vi "AE Events.vi"(8 "error in (no error)":errorcluster, 10 "Event In":dbl, 11 "Action":enum16{"Init", "Get Event", "Set Event"}(ring)) -> (0 "error out":errorcluster, 2 "Event Out":dbl)   [LabVIEW 2013, in "main.lvlib"]
uses:
  main.lvlib
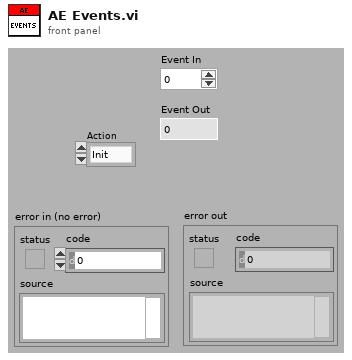
[diagram p1: front panel]
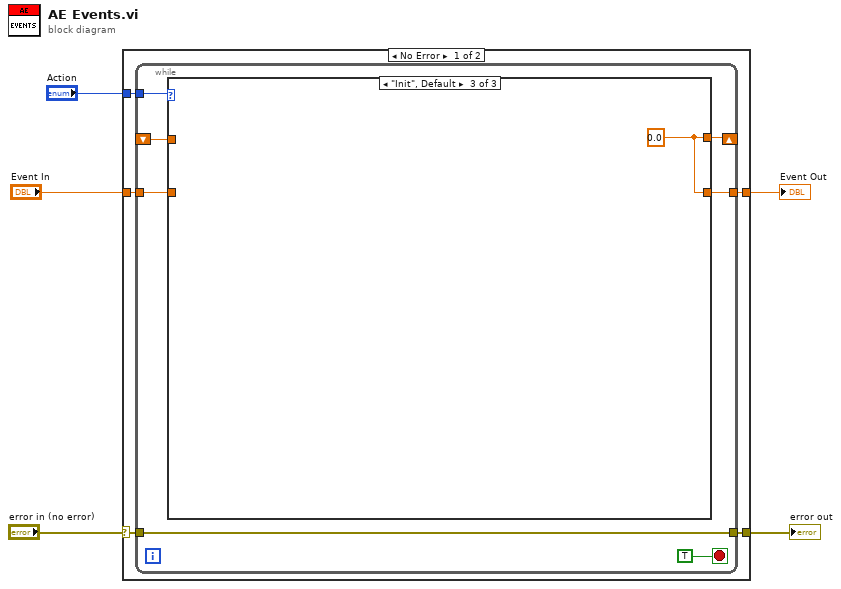
[diagram p0: block diagram]
diagram:
  n1 = case shown="No Error" "error in (no error)" {
    selector: "error in (no error)" -> [w7 w22]
    tunnel: "Action" -> [w10 _]
    tunnel: "Event In" -> [w9 w21]
    tunnel: [w8 w21] -> w3
    tunnel: [w6 w22] -> w1
    frame No Error {
      n2 = while {
        shift-right: [w15] -> _
        shift-left: _ -> [w16]
        tunnel: w10 -> [w17]
        tunnel: w9 -> [w14]
        tunnel: [w13] -> w8
        tunnel: w7 -> [w12]
        tunnel: [w12] -> w6
        stop <- TRUE stop-if-true
        n3 = case shown="\"Init\", Default" w17 {
          tunnel: [w18 w19 w20] -> w15
          tunnel: w16 -> [_ w19 _]
          tunnel: w14 -> [w18 _ _]
          tunnel: [w18 w19 w20] -> w13
          frame "Set Event" {
          }
          frame "Get Event" {
          }
          frame "Init", Default {
            w20 = 0.0 ("Event In")
          }
        }
      }
    }
    frame Error {
    }
  }
  "Event Out" <- w3
  "error out" <- w1
